vi "ConfParameters.vi"(2 "Configuration IN":T1={"Connection"={"Package Size"=1, "Sending Rate (ms)"=100, "TCP Port"=2055}, "General"={"StartJIL"=FALSE, "OpenFP"=TRUE}, "Authentication"={"user"="root", "Password"="kk", "UseAuthentication"=FALSE}}, 3 "Operatrion":string="load") -> (0 "error out":errorcluster, 1 "Configuration OUT":T1={"Connection"={"Package Size"=1, "Sending Rate (ms)"=100, "TCP Port"=2055}, "General"={"StartJIL"=FALSE, "OpenFP"=TRUE}, "Authentication"={"user"="root", "Password"="kk", "UseAuthentication"=FALSE}})   [LabVIEW 2010]
uses:
  <vilib>/Utility/xml.llb/Write to XML File(string).vi
  <vilib>/Utility/xml.llb/Read From XML File(string).vi
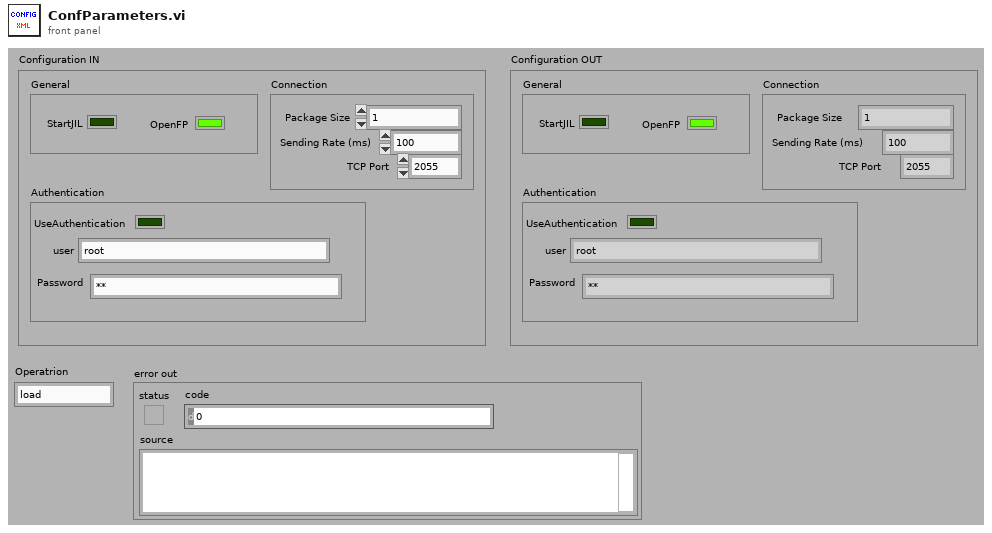
[diagram p1: front panel]
types:
  T1 = cluster{"Connection":cluster{"Package Size":u32, "Sending Rate (ms)":u32, "TCP Port":u32}, "General":cluster{"StartJIL":bool, "OpenFP":bool}, "Authentication":cluster{"user":string, "Password":string, "UseAuthentication":bool}}
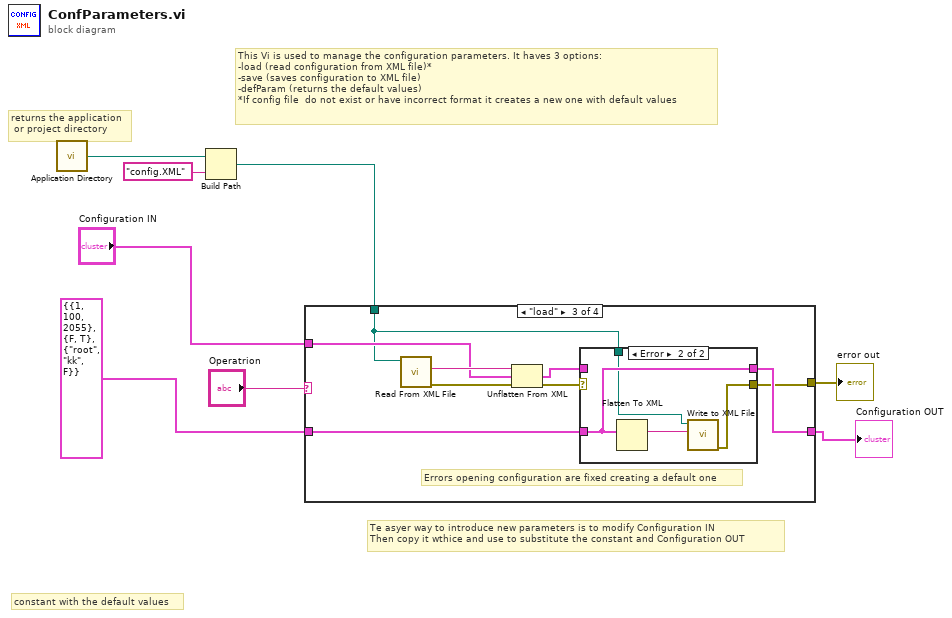
[diagram p0: block diagram]
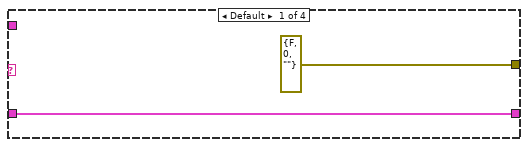
[diagram p2: hidden frame]
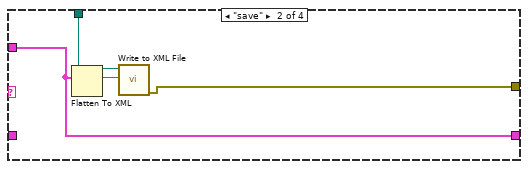
[diagram p3: hidden frame]
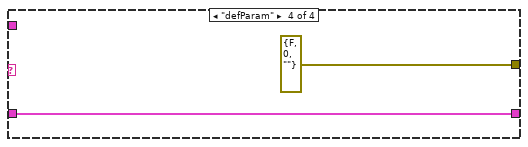
[diagram p5: hidden frame]
diagram:
  # "constant with the default values"
  # "Te asyer way to introduce new parameters is to modify Configuration IN\nThen copy it wthice and use to substitute the constant and Configuration OUT"
  # "returns the application\n or project directory"
  # "This Vi is used to manage the configuration parameters. It haves 3 options:\n-load (read configuration from XML file)*\n-save (saves configuration to XML file)\n-defParam (returns the default values)\n*If config file  do not exist or have incorrect format it creates a new one with default values"
  n1 = call <vilib>:"Application Directory.vi"() -> ("Application Directory"=w7:path)
  n2 = Build Path(base path=w7, name or relative path="config.XML") -> (appended path=w5:path)
  n3 = case shown="\"load\"" "Operatrion" {
    tunnel: T1 {"Connection"={"Package Size"=1, "Sending Rate (ms)"=100, "TCP Port"=2055}, "General"={"StartJIL"=FALSE, "OpenFP"=TRUE}, "Authentication"={"user"="root", "Password"="kk", "UseAuthentication"=FALSE}} ("Configuration IN") -> [w9 _ w16 w31]
    tunnel: [w9 w11 w19 w31] -> w1
    tunnel: w5 -> [_ w14 w15 _]
    tunnel: "Configuration IN" -> [_ w11 w22 _]
    tunnel: [errorcluster {"status"=FALSE, "code"=0, "source"=""} ("error out") w12 w17 errorcluster {"status"=FALSE, "code"=0, "source"=""} ("error out")] -> w3
    frame Default {
    }
    frame "save" {
      n4 = Flatten To XML(anything=w11) -> (xml string=w13:string)
      n5 = call-poly <vilib>:"Write to XML File.vi"("XML Input"=w13, "XML File Path"=w14) -> ("error out"=w12:errorcluster)  [unwired: 7 in, 2 out]
    }
    frame "load" {
      # "Errors opening configuration are fixed creating a default one"
      n6 = call-poly <vilib>:"Read From XML File.vi"("XML File Path"=w15) -> ("error out"=w21:errorcluster, "XML Elements"=w23:string)  [unwired: 8 in, 1 out]
      n7 = Unflatten From XML(xml string=w23, type=w22, error in (no error)=w21) -> (value=w18:T1, error out=w20:errorcluster)
      n8 = case shown="Error" w20 {
        selector: w20 -> [w24 _]
        tunnel: [w25 w29] -> w19
        tunnel: w18 -> [w25 _]
        tunnel: [w24 w26] -> w17
        tunnel: w16 -> [_ w29]
        tunnel: w15 -> [_ w27]
        frame No Error {
        }
        frame Error {
          n9 = Flatten To XML(anything=w29) -> (xml string=w28:string)
          n10 = call-poly <vilib>:"Write to XML File.vi"("XML Input"=w28, "XML File Path"=w27) -> ("error out"=w26:errorcluster)  [unwired: 7 in, 2 out]
        }
      }
    }
    frame "defParam" {
    }
  }
  "error out" <- w3
  "Configuration OUT" <- w1
